vi "Click Tester.vi"() -> ()   [LabVIEW 2017]
panel:
  in  "OK Button":bool
  out "Numeric":dbl
  in  "stop":bool
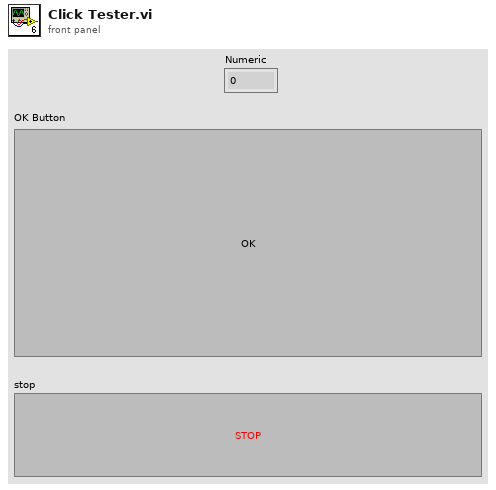
[diagram p1: front panel]
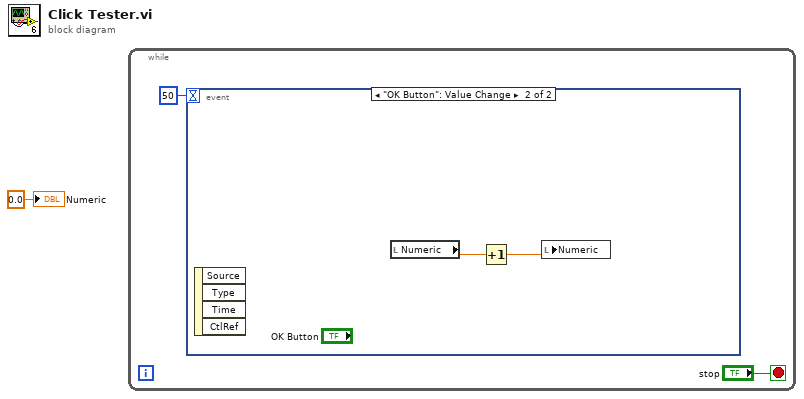
[diagram p0: block diagram]
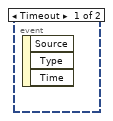
[diagram p2: hidden frame]
diagram:
  n1 = while {
    stop <- "stop" stop-if-true
    n2 = event shown="[1] \"OK Button\": Value Change" {
      selector: _ -> [_ _]
      dyn-events: _ -> [_ _]
      timeout: 50 -> [_ _]
      event Timeout {
        n3 = event-data() -> ()  [unwired: 1 in, 3 out]
      }
      event "OK Button": Value Change {
        n4 = event-data() -> ()  [unwired: 1 in, 4 out]
        n5 = local read "Numeric"() -> (w5:dbl)
        n6 = Increment(x=w5) -> (x+1=w4:dbl)
        n7 = local write "Numeric"(w4) -> ()
      }
    }
  }
  "Numeric" <- 0.0 ("Numeric")
